vi "format to JSON.vi"(0 "msg_type":enum16{"reply", "ack", "alert"}(ring), 5 "msg_parameter":T1(ring), 7 "element names":string[](array[string]), 9 "Values":dbl[](array[numeric]), 11 "error in":errorcluster) -> (4 "JSON string":string, 15 "error out":errorcluster)   [LabVIEW 2015]
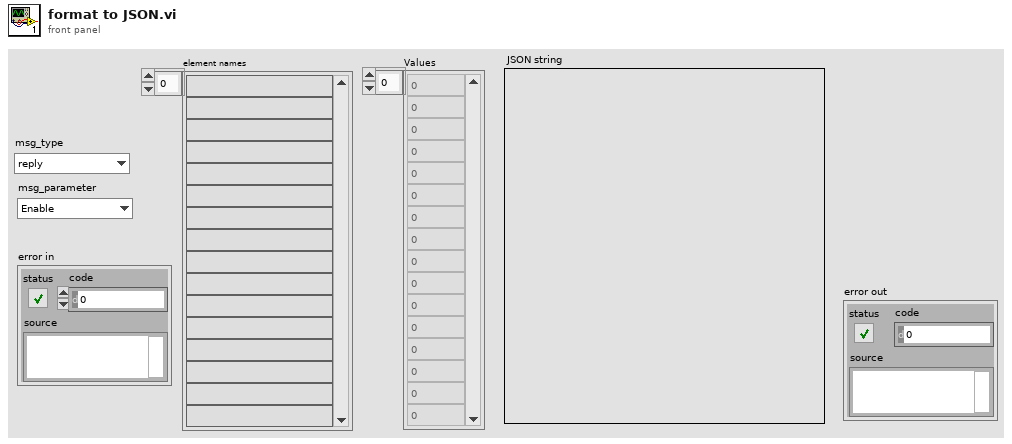
[diagram p1: front panel]
types:
  T1 = enum16{"Enable", "Status", "Vset", "Vmon", "Vswmax", "Imax", "Imon", "Trip"}
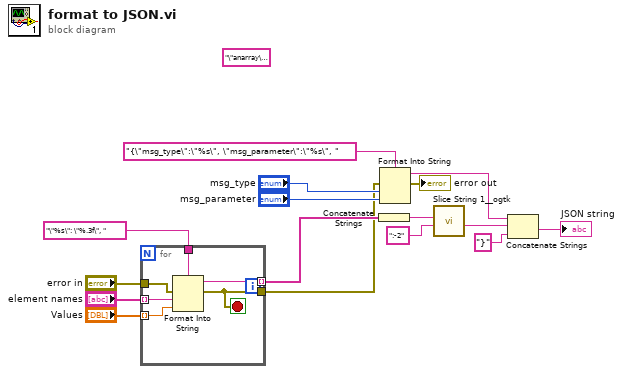
[diagram p0: block diagram]
diagram:
  (unwired) "\"anarray\": [\"var0\": \"0.00\", \"var1\": \"1.00\", \"var2\": \"2.00\", \"var3\": \"3.00\", \"var4\": \"4.00\", \"var5\": \"5.00\", \"var6\": \"6.00\", \"var7\": \"7.00\", \"var8\": \"8.00\", \"var9\": \"9.00\"]" ("JSON string 2")
  n1 = for {
    tunnel: [w22] -> w15 mode=indexing
    tunnel: "element names" -> [w21] mode=indexing
    tunnel: "Values" -> [w20] mode=indexing
    tunnel: [w18] -> w4
    tunnel: "\"%s\": \"%.3f\", " ("format string") -> [w19]
    tunnel: "error in" -> [w17]
    stop <- w18 stop-if-true
    n2 = Format Into String(format string=w19, error in=w17, w21, w20) -> (resulting string=w22:string, error out=w18:errorcluster)  [unwired: 1 in]
  }
  n3 = Concatenate Strings(w15) -> (w16:string)
  n4 = Format Into String(format string="{\"msg_type\":\"%s\", \"msg_parameter\":\"%s\", ", error in=w4, "msg_type", "msg_parameter") -> (resulting string=w9:string, error out=→"error out":errorcluster)  [unwired: 1 in]
  n5 = call <userlib>:"Slice String 1__ogtk.vi"("Subset (i:j)"=":-2", "String"=w16) -> ("Substring (String[i:j])"=w13:string)  [unwired: 7 in]
  n6 = Concatenate Strings(w9, w13, "}" ("Subset (i:j)")) -> (→"JSON string":string)
